vi "Aperture Server.vi"() -> ()   [LabVIEW 2018]
doc: "Use this VI to connect and control an unknown DC motor stage with the C-843. Select first if the connected stage is analog or PWM driven. The VI runs \"C843_Configuration_Setup.vi\" without moving any axis. It defines axis 1 to be \"DEFAULT_STAGE\" (analog) or \"DEFAULT_STAGE_P\" (PWM), which corresponds to no limit switches, no reference switch, and a position unit of 1 count. It reads the current velocity, the maximum allowed velocity, and the PID values of this stage type and sets the servo state to ON. Then it runs in a loop, reading the current position value, and giving the user the possibility to make relative moves in forward or backward direction, or to set velocity and PID values. Pressing the STOP button will send a STP command to the board, set the servo state to OFF and stop the VI."
uses:
  APERTURE EVENTS.ctl
  PI STAGE LIMITS.ctl
  PI APERTURE POSITION.ctl
  PI STAGE MAXIMUMS.ctl
  <vilib>/userdefined/High Color/IMAQdx.ctl
  <vilib>/vision/Image Controls.llb/Vision Info Type2.ctl
  <vilib>/Utility/miscctls.llb/LVMinMaxIncTypeDef.ctl
  <vilib>/Utility/Variable/NI_VariableUtilities.lvlib
  <vilib>/vision/NI_Vision_Development_Module.lvlib
  <vilib>/vision/driver/NI_Vision_Acquisition_Software.lvlib
panel:
  in  "ENABLE CAM":bool=TRUE
  in  "SET APERTURE":cluster{"Xm":dbl, "Ym":dbl} {"Ym" min=0.0 max=1.0 step=0.1 format="%.3f"; "Xm" min=0.0 max=12.5 step=0.1 format="%.3f"}
  in  "SET POSITION":T1 {"Yo" min=0.0 max=10.0 step=0.1 format="%.3f"; "Xo" min=0.0 max=12.5 step=0.1 format="%.3f"}
  out "APERTURE POSITION":cluster{"Xm":dbl, "Ym":dbl} {"Ym" format="%.3f"; "Xm" format="%.3f"}
  out "OBJECT POSITION":T1 {"Yo" format="%.3f"; "Xo" min=0.0 max=12.5 step=0.1 format="%.3f"}
  out "LIMITS ?":T2
  out "REFER?":T3
  out "ON TARG":T4
  out "SERVO?":T4
  out "HOMED":T5
  in  "INIT":bool=TRUE
  out "elements":T6[](array[typedef])
  in  "stop":bool
  in  "CLEAR ERRORS":bool
  out "PROCESS":string
  out "Identification":string
  out "Line Profile Graph":u8[](graph) caption="Line Profile"
  in  "Calibration Axis Info (Aperture Calibration)":T7={"Origin Pixel"={"X"=227.0, "Y"=1000.0}, "X Axis Pixel"={"X"=276.9972, "Y"=1000.52985}, "Axis Reference"=1} {"Axis Reference" items=["Direct", "Indirect"]}
  out "Image":T8(plugin-control)
  in  "PIXEL CALIBRATION":T9={"XSTEP SIZE"=5.7150000000000025, "YSTEP SIZE"=6.25, "UNITS"=2} {"UNITS" items=["Undefined", "Angstroms", "Microns"]; "YSTEP SIZE" format="%_4g"; "XSTEP SIZE" format="%_4g"}
  in  "BCG":T10={"BRIGHT"=150.0, "CONTRAST"=30.0, "GAMMA"=1.0} {"GAMMA" format="%_3f"}
  out "x-y":u16
  out "x*y":dbl
  in  "Tab Control":enum32{" SHIFTING", "SETTINGS", "RANGE"}(tab)
  out "HOMED":bool
  in  "AXIS":u16(ring) items=["1", "2", "3", "4"]
  in  "HOME LIMIT":enum16{"NEGATIVE", "POSITIVE"}(ring)
  in  "Stop":bool
  in  "STEP":dbl=1.0 min=0.0 max=1.0 step=0.1 format="%.4f"
  in  "OUT (+)":bool
  in  "IN (-)":bool
  in  "HOME":bool
  in  "HOME AXES":enum16{"1 & 2", "3 & 4"}(ring)
  out "Axis moving?":bool[](array[boolean])
  out "READY AXES":string[](array[string])
  in  "SERVO PID":cluster{"P":dbl, "I":dbl, "D":dbl}={"P"=140.0, "I"=14.0, "D"=300.0} {"P" format="%#.6f"; "I" format="%#.6f"; "D" format="%#.6f"}
  in  "STARTUP":T6[](array[typedef])=[enum."INIT PI CONTROLLER", enum."READ STAGE LIMIT SWITCHES ", enum."READ RON?", enum."SET SERVO MOTORS ON", enum."HOMED ?", enum."READ MIN POSITION: LIMIT OR SOFT"]
  in  "VELOCITY":dbl=10.0 format="%#.0p"
  out "STAGE MIN CLUSTER":T11 {"Xo MAX" format="%.6f"; "Xm MAX" format="%.6f"; "Ym MAX" format="%.6f"; "Yo MAX" format="%.6f"}
  out "STAGE MAX CLUSTER":T12 {"Xo MAX" format="%.6f"; "Xm MAX" format="%.6f"; "Ym MAX" format="%.6f"; "Yo MAX" format="%.6f"}
  in  "error in":errorcluster
  out "error out":errorcluster
  # "Radius 5.75cm for top element to\n centre optical element"
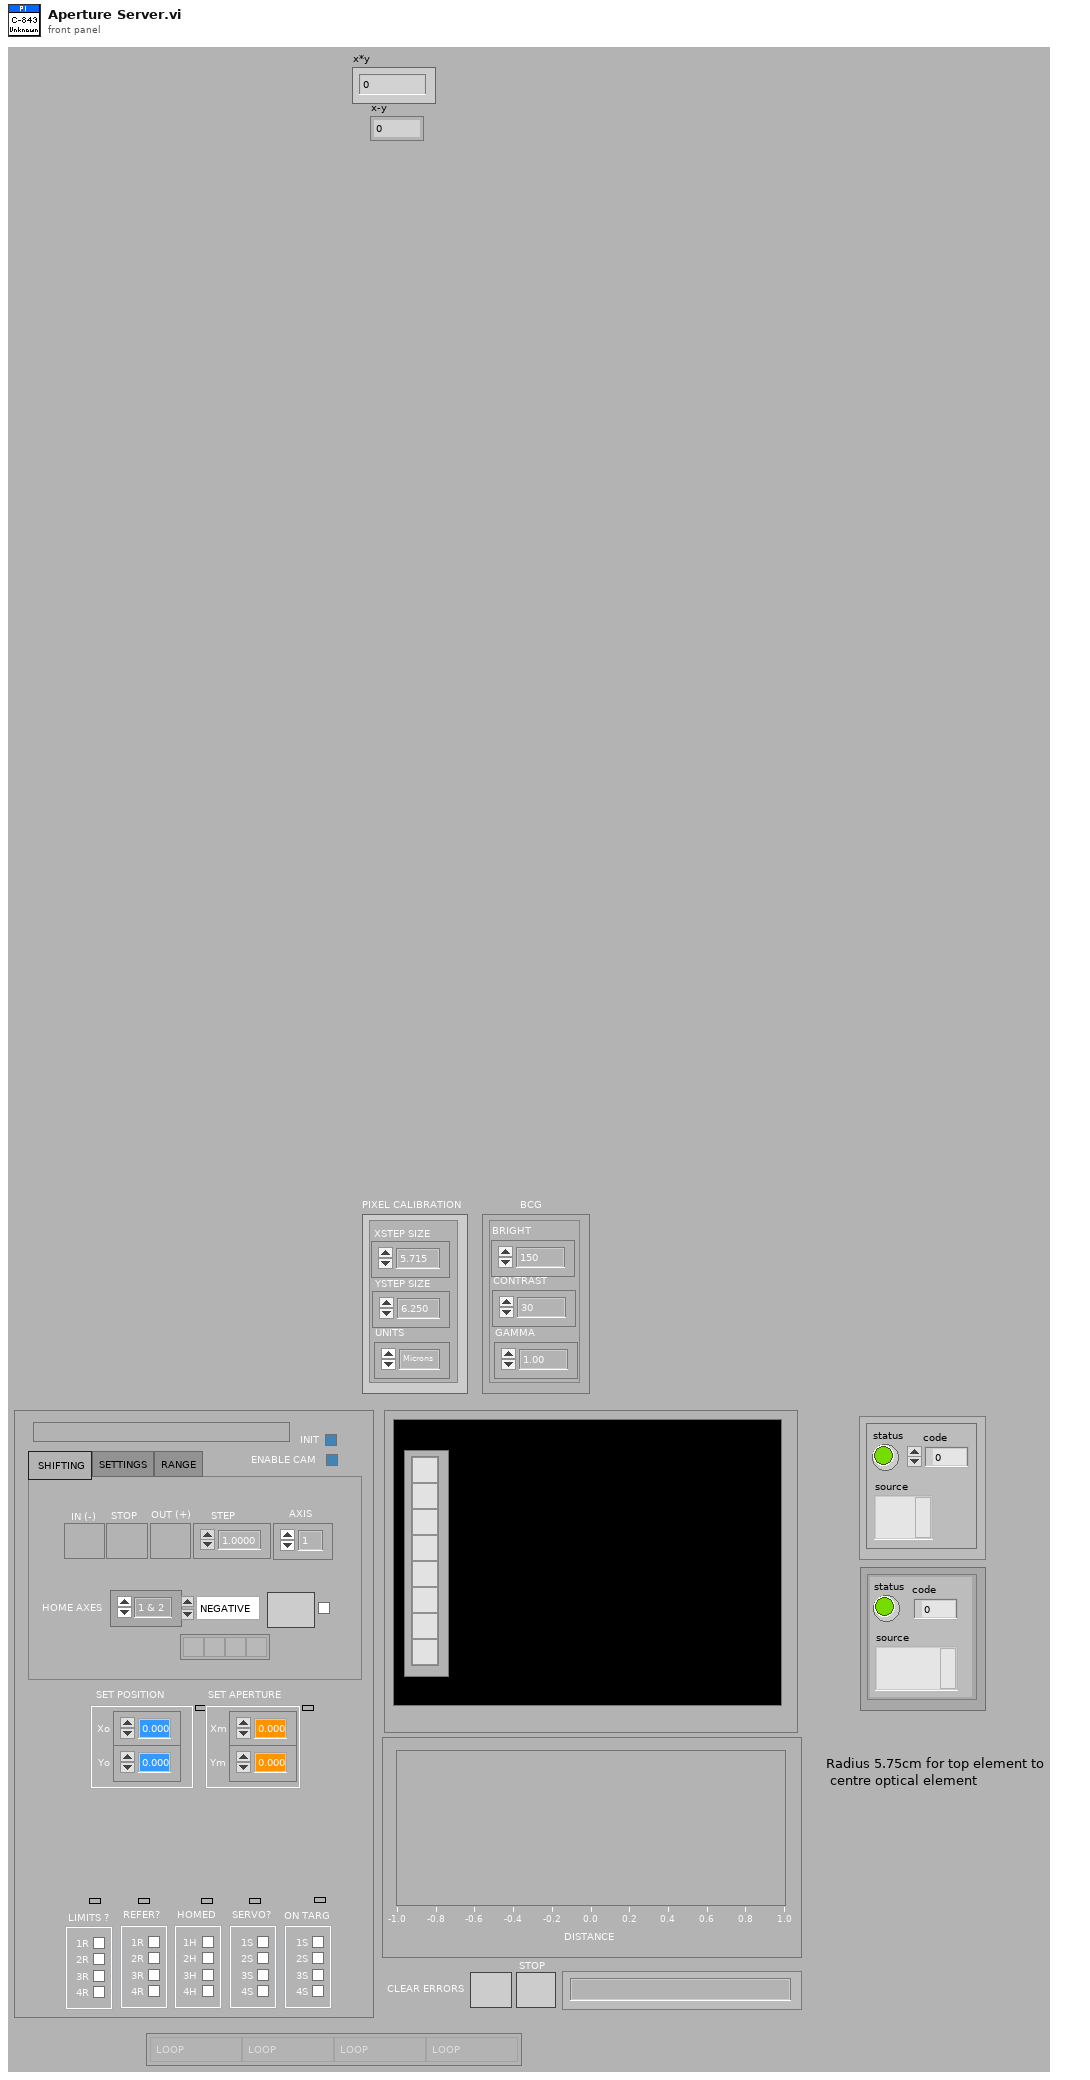
[diagram p1: front panel]
types:
  T1 = typedef "PI APERTURE POSITION.ctl" = cluster{"Xo":dbl, "Yo":dbl}
  T2 = typedef "PI STAGE LIMITS.ctl" = cluster{"1R":bool, "2R":bool, "3R":bool, "4R":bool}
  T3 = cluster{"1R":bool, "2R":bool, "3R":bool, "4R":bool}
  T4 = cluster{"1S":bool, "2S":bool, "3S":bool, "4S":bool}
  T5 = cluster{"1H":bool, "2H":bool, "3H":bool, "4H":bool}
  T6 = typedef "APERTURE EVENTS.ctl" = enum16{"LOOP", "INIT PI CONTROLLER", "WAIT FOR READY", "CLR ERRORS", "GOTO LIMIT", "HOMED ?", "READ MIN POSITION: LIMIT OR SOFT", "READ STAGE LIMIT SWITCHES ", "READ RON?", "GOTO POSITION", "SET POSITION", "GOTO LEFT", "GOTO RIGHT", "READ POSITION", "READ SERVO SETTINGS", "SET SERVO PID", "SET SERVO MOTORS ON", "SET VELOCITIES"}
  T7 = cluster{"Origin Pixel":cluster{"X":sgl, "Y":sgl}, "X Axis Pixel":cluster{"X":sgl, "Y":sgl}, "Axis Reference":u32}
  T8 = typedef "IMAQ Image.ctl" = refnum<image>
  T9 = cluster{"XSTEP SIZE":dbl, "YSTEP SIZE":dbl, "UNITS":u16}
  T10 = cluster{"BRIGHT":dbl, "CONTRAST":dbl, "GAMMA":dbl}
  T11 = typedef "PI STAGE MAXIMUMS.ctl" = cluster{"Xo MAX":dbl, "Xm MAX":dbl, "Yo MAX":dbl, "Ym MAX":dbl}
  T12 = cluster{"Xo MAX":dbl, "Xm MAX":dbl, "Yo MAX":dbl, "Ym MAX":dbl}
  T13 = typedef "IMAQdx.ctl" = refnum<k21>
  T14 = typedef "Vision Info Type2.ctl" = u32
  T15 = cluster{"Global Rectangle":i32[], "Contours":cluster{"Contour Type":u32, "ROI Type":u32, "Points":i32[]}[]}
  T16 = cluster{"Boolean":bool, "Boolean":bool, "Boolean":bool, "Boolean":bool}
  T17 = typedef "LVMinMaxIncTypeDef.ctl" = cluster{"Minimum":dbl, "Maximum":dbl, "Increment":dbl}
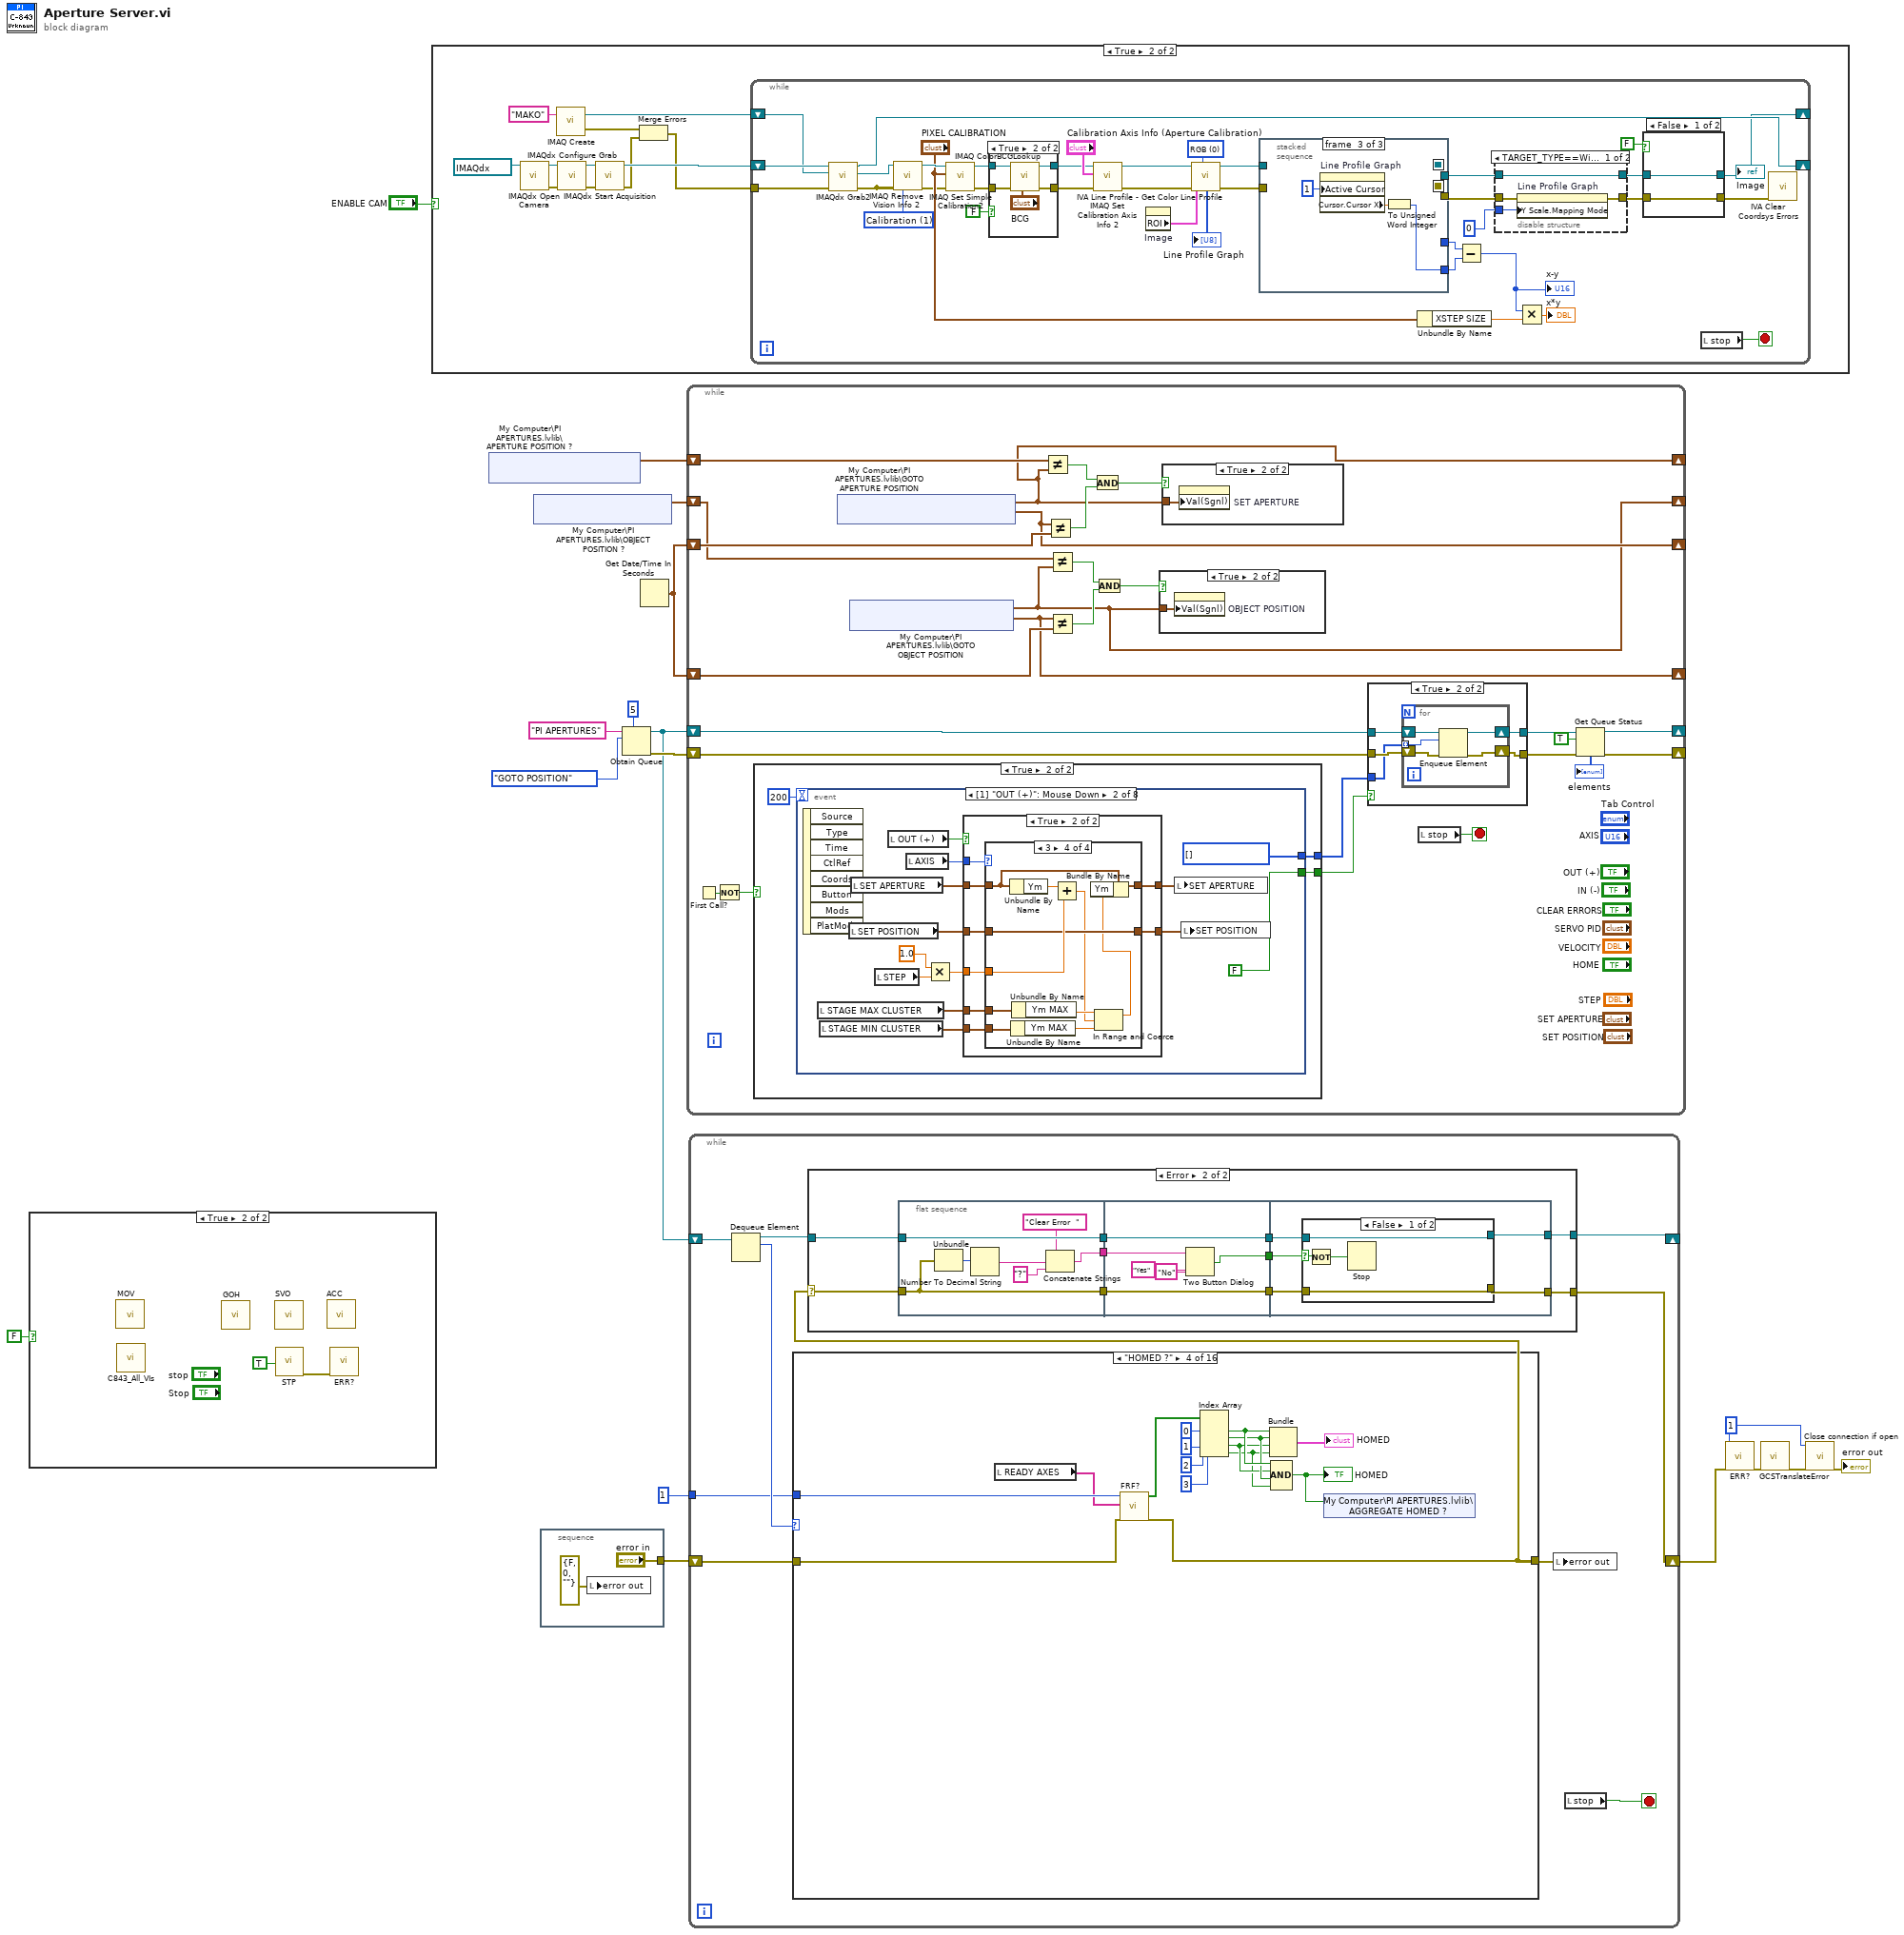
[diagram p0: block diagram]
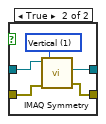
[diagram p3: hidden frame]
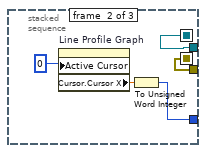
[diagram p6: hidden frame]
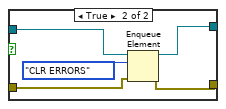
[diagram p10: hidden frame]
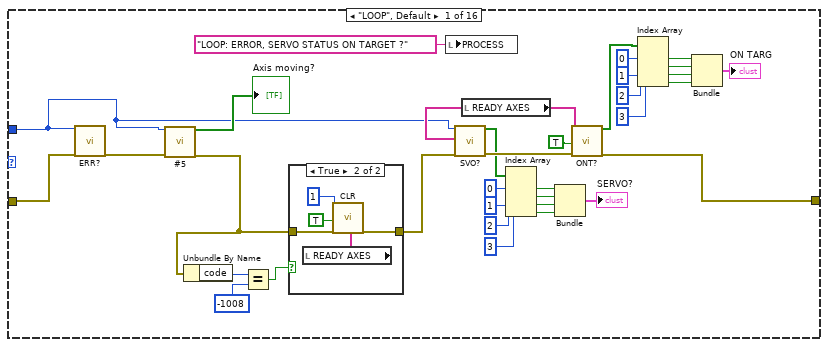
[diagram p11: hidden frame]
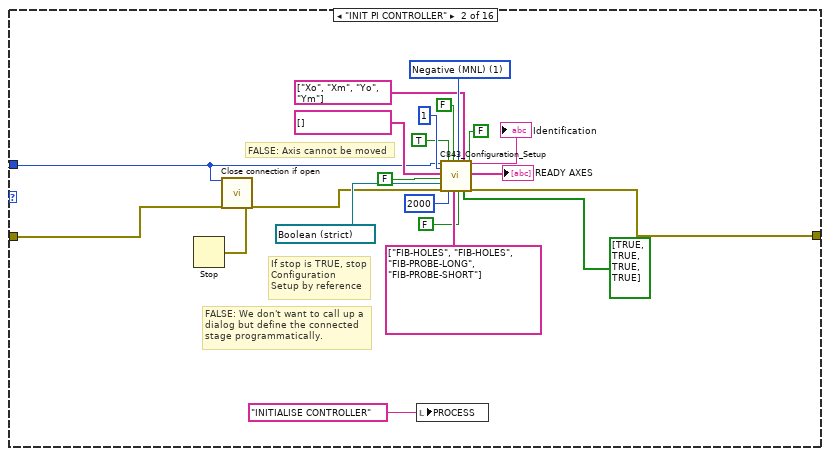
[diagram p13: hidden frame]
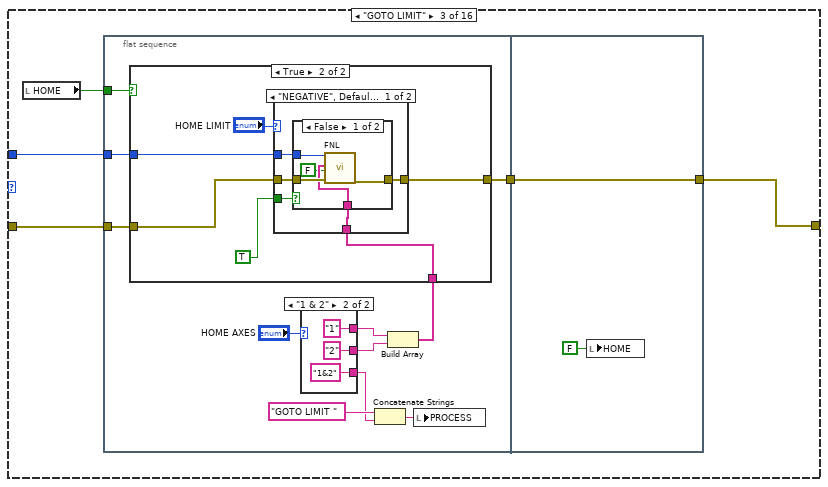
[diagram p14: hidden frame]
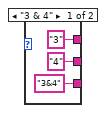
[diagram p15: hidden frame]
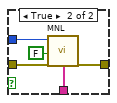
[diagram p17: hidden frame]
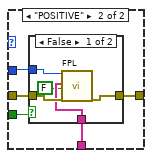
[diagram p18: hidden frame]
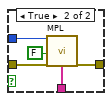
[diagram p19: hidden frame]
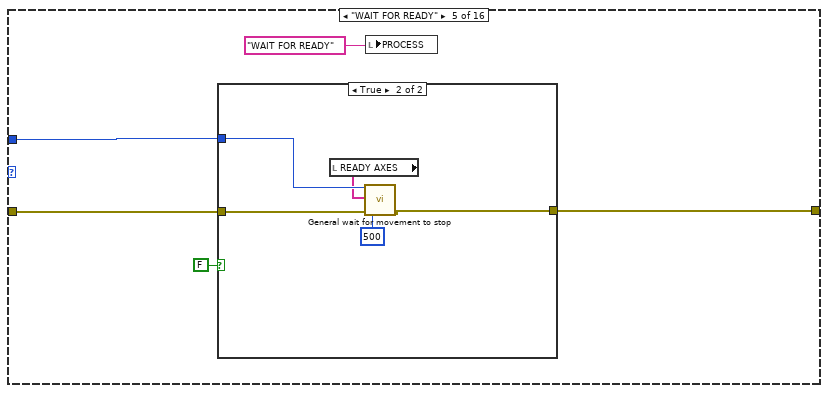
[diagram p20: hidden frame]
diagram:
  w5 = 1 ("System no.")
  n1 = case shown="True" FALSE {
    frame False {
    }
    frame True {
      n2 = call "MOV.vi"() -> ()  [unwired: 5 in, 15 out]
      n3 = call "C843_All_VIs.vi"() -> ()  [unwired: 1 in]
      n4 = call "GOH.vi"() -> ()  [unwired: 5 in, 15 out]
      n5 = call "SVO.vi"() -> ()  [unwired: 5 in, 15 out]
      n6 = call "STP.vi"("All axes?"=TRUE) -> ("error out"=w19:errorcluster)  [unwired: 4 in, 14 out]
      n7 = call "ACC.vi"() -> ()  [unwired: 6 in, 14 out]
      n8 = call "ERR?.vi"("error in"=w19) -> ()  [unwired: 1 in, 18 out]
    }
  }
  n9 = case shown="True" "ENABLE CAM" {
    frame False {
    }
    frame True {
      n10 = call <vilib>:"IMAQdx Open Camera.vi"("Session In"=T13 "MAKO") -> ("error out"=w27:errorcluster, "Session Out"=w29:T13)  [unwired: 9 in]
      n11 = call "IMAQ Create"("Image Name"="MAKO") -> ("New Image"=w23:T8, "error out"=w22:errorcluster)  [unwired: 4 in]
      n12 = call <vilib>:"IMAQdx Configure Grab.vi"("error in"=w27, "Session In"=w29) -> ("error out"=w26:errorcluster, "Session Out"=w28:T13)  [unwired: 8 in]
      n13 = call <vilib>:"IMAQdx Start Acquisition.vi"("error in"=w26, "Session In"=w28) -> ("error out"=w21:errorcluster, "Session Out"=w24:T13)  [unwired: 8 in]
      n14 = Merge Errors(w22, w21) -> (w20:errorcluster)
      n15 = while {
        tunnel: w20 -> [w43]
        shift-right: [w39] -> _
        shift-left: w24 -> [w42]
        shift-right: [w35] -> _
        shift-left: w23 -> [w38]
        stop <- w37 stop-if-true
        w63 = u16 0 items=["RGB", "HSL", "HSV", "HSI"] ("Color Mode")
        w66 = T14 1 items=["Any", "Calibration", "Overlay", "Grayscale Template", "Color Template", "Geometric Template", "Custom Data", "Golden Template", "Geometric Template 2", "Contour Data", "Camera Model"] ("Vision Info")
        n16 = call <vilib>:"IMAQdx Grab2.vi"("error in"=w43, "Image In"=w38, "Session In"=w42) -> ("error out"=w40:errorcluster, "Image Out"=w41:T8, "Session Out"=w39:T13)  [unwired: 5 in, 1 out]
        n17 = call "IMAQ Remove Vision Info 2"("error in (no error)"=w40, "Vision Info"=w66, "Image"=w41) -> ("Image Out"=w65:T8)  [unwired: 8 out]
        n18 = call "IMAQ Set Simple Calibration2"("error in (no error)"=w40, "Pixel Distances"="PIXEL CALIBRATION", "Image"=w65) -> ("error out"=w56:errorcluster, "Calibration Template Image"=w58:T8)  [unwired: 2 in, 5 out]
        n19 = case shown="True" FALSE {
          tunnel: w58 -> [w75 w80]
          tunnel: [w75 w79] -> w57
          tunnel: w56 -> [w74 w78]
          tunnel: [w74 w77] -> w55
          frame False {
          }
          frame True {
            n20 = call "IMAQ ColorBCGLookup"("Green BCG Values"="BCG", "error in (no error)"=w78, "Image Src"=w80) -> ("error out"=w77:errorcluster, "Image Dst Out"=w79:T8)  [unwired: 4 in, 3 out]
          }
        }
        n21 = call-poly "IMAQ Set Calibration Axis Info 2"("error in (no error)"=w55, "Calibration Axis Info"="Calibration Axis Info (Aperture Calibration)", "Calibration Template Image In"=w57) -> ("error out"=w61:errorcluster, "Calibration Template Image Out"=w62:T8)  [unwired: 7 out]
        n22 = property on="Image" class="ImageControl"() -> ("ROI"=w54:T15)  [unwired: 2 in, 2 out]
        n23 = call <vilib>:"IVA Line Profile - Get Color Line Profile.vi"("Color Mode"=w63, "error in (no error)"=w61, "ROI Descriptor"=w54, "Image In"=w62) -> ("error out"=w50:errorcluster, "Green or Sat Pixels"=→"Line Profile Graph":u8[], "Image Out"=w52:T8)  [unwired: 5 out]
        n24 = stacked-sequence {
          seq-local: [w82 _ _] -> [_ w84 _]
          seq-local: [w81 _ _] -> [_ w83 _]
          tunnel: w52 -> [w82 _ _]
          tunnel: w50 -> [w81 _ _]
          tunnel: [_ w84 _] -> w53
          tunnel: [_ w83 _] -> w51
          tunnel: [_ w85 _] -> w49
          tunnel: [_ _ w88] -> w48
          frame #0 {
          }
          frame #1 {
            n25 = property on="Line Profile Graph" class="WFGraph (strict)"("Active Cursor"=u32 0) -> ("Cursor.Cursor X"=w86:dbl)  [unwired: 2 in, 2 out]
            n26 = To Unsigned Word Integer(number=w86) -> (unsigned 16bit integer=w85:u16)
          }
          frame #2 {
            n27 = property on="Line Profile Graph" class="WFGraph (strict)"("Active Cursor"=u32 1) -> ("Cursor.Cursor X"=w89:dbl)  [unwired: 2 in, 2 out]
            n28 = To Unsigned Word Integer(number=w89) -> (unsigned 16bit integer=w88:u16)
          }
        }
        n29 = Unbundle By Name("PIXEL CALIBRATION") -> ("XSTEP SIZE"=w45:dbl)
        n30 = Subtract(x=w49, y=w48) -> (x-y=w47:u16)
        "x-y" <- w47
        n31 = disable-structure "Conditional Disable Structure" shown="TARGET_TYPE==Windows" {
          disable-tunnel: w51 -> [w94 w95]
          disable-tunnel: [w93 w95] -> w33
          disable-tunnel: w53 -> [w92 w96]
          disable-tunnel: [w92 w96] -> w34
          disable-tunnel: u8 0 ("Y Scale.Mapping Mode") -> [w91 _]
          frame condition #0 (active) {
            n32 = property on="Line Profile Graph" class="WFGraph (strict)"(error in=w94, "Y Scale.Mapping Mode"=w91) -> (error out=w93:errorcluster)  [unwired: 1 in, 1 out]
          }
          frame condition #1 {
          }
        }
        n33 = Multiply(x=w47, y=w45) -> (x*y=→"x*y":dbl)
        n34 = case shown="False" FALSE {
          tunnel: [w68 w73] -> w35
          tunnel: w34 -> [w68 w72]
          tunnel: w33 -> [w67 w70]
          tunnel: [w67 w69] -> w32
          frame False {
          }
          frame True {
            w71 = u32 1 items=["Horizontal", "Vertical", "Central", "1st Diagonal", "2nd Diagonal"] ("Type of Symmetry")
            n35 = call "IMAQ Symmetry"("error in (no error)"=w70, "Type of Symmetry"=w71, "Image Src"=w72) -> ("error out"=w69:errorcluster, "Image Dst Out"=w73:T8)  [unwired: 2 in]
          }
        }
        "Image" <- w35
        n36 = local read "stop"() -> (w37:bool)
        n37 = call <vilib>:"IVA Clear Coordsys Errors.vi"("error in (no error)"=w32) -> ()  [unwired: 10 in, 1 out]
      }
    }
  }
  n38 = shared-variable "My Computer\\PI APERTURES.lvlib\\APERTURE POSITION ?"() -> (w3:cluster{"Xm":dbl, "Ym":dbl})  [unwired: 1 in, 2 out]
  n39 = shared-variable "My Computer\\PI APERTURES.lvlib\\OBJECT POSITION ?"() -> (w2:cluster{"Xm":dbl, "Ym":dbl})  [unwired: 1 in, 2 out]
  n40 = stacked-sequence {
    tunnel: ["error in"] -> w6
    frame #0 {
      n41 = local write "error out"(errorcluster {"status"=FALSE, "code"=0, "source"=""} ("error in")) -> ()
    }
  }
  n42 = Obtain Queue(max queue size (-1, unlimited)=5, name (unnamed)="PI APERTURES", element data type=APERTURE_EVENTS."GOTO POSITION") -> (queue out=w11:refnum<queue>, error out=w12:errorcluster)  [unwired: 2 in, 1 out]
  n43 = Get Date/Time In Seconds() -> (seconds since 1Jan1904=w4:timestamp)
  n44 = while {
    shift-right: [w119] -> _
    shift-left: w11 -> [w115]
    shift-right: [w117] -> _
    shift-left: w12 -> [w114]
    shift-right: [w111] -> _
    shift-left: w4 -> [w112]
    shift-right: [w109] -> _
    shift-left: w4 -> [w110]
    shift-right: [w100] -> _
    shift-left: w3 -> [w105]
    shift-right: [w99] -> _
    shift-left: w2 -> [w104]
    stop <- w121 stop-if-true
    n45 = First Call?() -> (First Call?: T/F=w123:bool)
    n46 = Not(x=w123) -> (.not. x?=w122:bool)
    n47 = case shown="True" w122 {
      tunnel: [w133 w141] -> w125
      tunnel: [TRUE w140] -> w124
      frame False {
        n48 = local write "HOME AXES"(enum16{"1 & 2", "3 & 4"}."1 & 2" ("HOME AXES")) -> ()
        n49 = local write "HOME LIMIT"(enum16{"NEGATIVE", "POSITIVE"}."NEGATIVE" ("HOME LIMIT")) -> ()
        n50 = Delete From Array(array="STARTUP", length=1, index=0) -> (array with subset deleted=w132:T6[])  [unwired: 1 out]
        n51 = case shown="False" "INIT" {
          tunnel: [w138 w139] -> w133
          tunnel: w132 -> [w138 _]
          tunnel: "STARTUP" -> [_ w139]
          frame False {
          }
          frame True {
          }
        }
        "PROCESS" <- "" ("PROCESS")
      }
      frame True {
        n52 = event shown="[1] \"OUT (+)\": Mouse Down" {
          selector: _ -> [_ _ _ _ _ _ _ _]
          dyn-events: _ -> [_ _ _ _ _ _ _ _]
          timeout: 200 -> [_ _ _ _ _ _ _ _]
          tunnel: [w144 w149 w216 w280 w282 w284 w285 w288] -> w141
          tunnel: [TRUE FALSE ("HOMED") FALSE ("HOMED") w279 TRUE TRUE TRUE TRUE] -> w140
          event Timeout {
            w144 = T6[] [enum."LOOP", enum."READ POSITION", enum."HOMED ?"] items=["LOOP", "INIT PI CONTROLLER", "WAIT FOR READY", "CLR ERRORS", "GOTO LIMIT", "HOMED ?", "READ MIN POSITION: LIMIT OR SOFT", "READ STAGE LIMIT SWITCHES ", "READ RON?", "GOTO POSITION", "SET POSITION", "GOTO LEFT", "GOTO RIGHT", "READ POSITION", "READ SERVO SETTINGS", "SET SERVO PID", "SET SERVO MOTORS ON", "SET VELOCITIES"]
            n53 = event-data() -> ()  [unwired: 1 in, 3 out]
            n54 = call <vilib>:"Flush Shared Variable Data.vi"() -> ()  [unwired: 11 in, 1 out]
          }
          event "OUT (+)": Mouse Down {
            w149 = T6[] [] items=["LOOP", "INIT PI CONTROLLER", "WAIT FOR READY", "CLR ERRORS", "GOTO LIMIT", "HOMED ?", "READ MIN POSITION: LIMIT OR SOFT", "READ STAGE LIMIT SWITCHES ", "READ RON?", "GOTO POSITION", "SET POSITION", "GOTO LEFT", "GOTO RIGHT", "READ POSITION", "READ SERVO SETTINGS", "SET SERVO PID", "SET SERVO MOTORS ON", "SET VELOCITIES"]
            n55 = event-data() -> ()  [unwired: 1 in, 8 out]
            n56 = local read "STAGE MAX CLUSTER"() -> (w145:T12)
            n57 = local read "STAGE MIN CLUSTER"() -> (w146:T11)
            n58 = local read "SET POSITION"() -> (w155:T1)
            n59 = local read "SET APERTURE"() -> (w156:cluster{"Xm":dbl, "Ym":dbl})
            n60 = local read "STEP"() -> (w154:dbl)
            n61 = local read "OUT (+)"() -> (w147:bool)
            n62 = local read "AXIS"() -> (w153:u16)
            n63 = Multiply(x=1.0, y=w154) -> (x*y=w157:dbl)
            n64 = case shown="True" w147 {
              tunnel: w157 -> [_ w167]
              tunnel: w156 -> [w159 w166]
              tunnel: w155 -> [w158 w165]
              tunnel: w153 -> [_ w164]
              tunnel: [w158 w163] -> w151
              tunnel: [w159 w162] -> w150
              tunnel: w146 -> [_ w161]
              tunnel: w145 -> [_ w160]
              frame False {
              }
              frame True {
                n65 = case shown="3" w164 {
                  tunnel: w165 -> [w176 w187 w198 w207]
                  tunnel: w166 -> [w174 w188 w196 w210]
                  tunnel: w167 -> [w177 w185 w199 w208]
                  tunnel: [w175 w187 w197 w207] -> w163
                  tunnel: [w174 w186 w196 w209] -> w162
                  tunnel: w161 -> [w172 w181 w192 w201]
                  tunnel: w160 -> [w173 w182 w193 w202]
                  frame 0, Default {
                    n66 = Unbundle By Name(w172) -> ("Xo MAX"=w170:dbl)
                    n67 = Unbundle By Name(w173) -> ("Xo MAX"=w171:dbl)
                    n68 = Unbundle By Name(w176) -> ("Xo"=w178:dbl)
                    n69 = Add(x=w178, y=w177) -> (x+y=w169:dbl)
                    n70 = In Range and Coerce(upper limit=w171, x=w169, lower limit=w170) -> (coerced(x)=w168:dbl)  [unwired: 1 out]
                    n71 = Bundle By Name(cluster=w176, "Xo"=w168) -> (w175:T1)
                  }
                  frame 1 {
                    n72 = Unbundle By Name(w188) -> ("Xm"=w189:dbl)
                    n73 = Unbundle By Name(w181) -> ("Xm MAX"=w183:dbl)
                    n74 = Unbundle By Name(w182) -> ("Xm MAX"=w184:dbl)
                    n75 = Add(x=w189, y=w185) -> (x+y=w180:dbl)
                    n76 = In Range and Coerce(upper limit=w184, x=w180, lower limit=w183) -> (coerced(x)=w179:dbl)  [unwired: 1 out]
                    n77 = Bundle By Name(cluster=w188, "Xm"=w179) -> (w186:cluster{"Xm":dbl, "Ym":dbl})
                  }
                  frame 2 {
                    n78 = Unbundle By Name(w192) -> ("Yo MAX"=w195:dbl)
                    n79 = Unbundle By Name(w193) -> ("Yo MAX"=w194:dbl)
                    n80 = Unbundle By Name(w198) -> ("Yo"=w200:dbl)
                    n81 = Add(x=w200, y=w199) -> (x+y=w191:dbl)
                    n82 = In Range and Coerce(upper limit=w194, x=w191, lower limit=w195) -> (coerced(x)=w190:dbl)  [unwired: 1 out]
                    n83 = Bundle By Name(cluster=w198, "Yo"=w190) -> (w197:T1)
                  }
                  frame 3 {
                    n84 = Unbundle By Name(w210) -> ("Ym"=w211:dbl)
                    n85 = Unbundle By Name(w201) -> ("Ym MAX"=w206:dbl)
                    n86 = Unbundle By Name(w202) -> ("Ym MAX"=w205:dbl)
                    n87 = Add(x=w211, y=w208) -> (x+y=w204:dbl)
                    n88 = In Range and Coerce(upper limit=w205, x=w204, lower limit=w206) -> (coerced(x)=w203:dbl)  [unwired: 1 out]
                    n89 = Bundle By Name(cluster=w210, "Ym"=w203) -> (w209:cluster{"Xm":dbl, "Ym":dbl})
                  }
                }
              }
            }
            n90 = local write "SET APERTURE"(w150) -> ()
            n91 = local write "SET POSITION"(w151) -> ()
          }
          event "IN (-)": Mouse Down {
            w216 = T6[] [] items=["LOOP", "INIT PI CONTROLLER", "WAIT FOR READY", "CLR ERRORS", "GOTO LIMIT", "HOMED ?", "READ MIN POSITION: LIMIT OR SOFT", "READ STAGE LIMIT SWITCHES ", "READ RON?", "GOTO POSITION", "SET POSITION", "GOTO LEFT", "GOTO RIGHT", "READ POSITION", "READ SERVO SETTINGS", "SET SERVO PID", "SET SERVO MOTORS ON", "SET VELOCITIES"]
            n92 = event-data() -> ()  [unwired: 1 in, 7 out]
            n93 = local read "STAGE MAX CLUSTER"() -> (w212:T12)
            n94 = local read "STAGE MIN CLUSTER"() -> (w213:T11)
            n95 = local read "SET POSITION"() -> (w222:T1)
            n96 = local read "SET APERTURE"() -> (w223:cluster{"Xm":dbl, "Ym":dbl})
            n97 = local read "STEP"() -> (w221:dbl)
            n98 = local read "OUT (+)"() -> (w214:bool)
            n99 = local read "AXIS"() -> (w220:u16)
            n100 = Multiply(x=-1.0, y=w221) -> (x*y=w224:dbl)
            n101 = case shown="True" w214 {
              tunnel: w224 -> [_ w234]
              tunnel: w223 -> [w226 w233]
              tunnel: w222 -> [w225 w232]
              tunnel: w220 -> [_ w231]
              tunnel: [w225 w230] -> w218
              tunnel: [w226 w229] -> w217
              tunnel: w213 -> [_ w228]
              tunnel: w212 -> [_ w227]
              frame False {
              }
              frame True {
                n102 = case shown="3" w231 {
                  tunnel: w232 -> [w243 w254 w265 w274]
                  tunnel: w233 -> [w241 w255 w263 w277]
                  tunnel: w234 -> [w244 w252 w266 w275]
                  tunnel: [w242 w254 w264 w274] -> w230
                  tunnel: [w241 w253 w263 w276] -> w229
                  tunnel: w228 -> [w239 w248 w259 w268]
                  tunnel: w227 -> [w240 w249 w260 w269]
                  frame 0, Default {
                    n103 = Unbundle By Name(w240) -> ("Xo MAX"=w238:dbl)
                    n104 = Unbundle By Name(w239) -> ("Xo MAX"=w237:dbl)
                    n105 = Unbundle By Name(w243) -> ("Xo"=w245:dbl)
                    n106 = Add(x=w245, y=w244) -> (x+y=w236:dbl)
                    n107 = In Range and Coerce(upper limit=w238, x=w236, lower limit=w237) -> (coerced(x)=w235:dbl)  [unwired: 1 out]
                    n108 = Bundle By Name(cluster=w243, "Xo"=w235) -> (w242:T1)
                  }
                  frame 1 {
                    n109 = Unbundle By Name(w255) -> ("Xm"=w256:dbl)
                    n110 = Unbundle By Name(w248) -> ("Xm MAX"=w250:dbl)
                    n111 = Unbundle By Name(w249) -> ("Xm MAX"=w251:dbl)
                    n112 = Add(x=w256, y=w252) -> (x+y=w247:dbl)
                    n113 = In Range and Coerce(upper limit=w251, x=w247, lower limit=w250) -> (coerced(x)=w246:dbl)  [unwired: 1 out]
                    n114 = Bundle By Name(cluster=w255, "Xm"=w246) -> (w253:cluster{"Xm":dbl, "Ym":dbl})
                  }
                  frame 2 {
                    n115 = Unbundle By Name(w259) -> ("Yo MAX"=w262:dbl)
                    n116 = Unbundle By Name(w260) -> ("Yo MAX"=w261:dbl)
                    n117 = Unbundle By Name(w265) -> ("Yo"=w267:dbl)
                    n118 = Add(x=w267, y=w266) -> (x+y=w258:dbl)
                    n119 = In Range and Coerce(upper limit=w261, x=w258, lower limit=w262) -> (coerced(x)=w257:dbl)  [unwired: 1 out]
                    n120 = Bundle By Name(cluster=w265, "Yo"=w257) -> (w264:T1)
                  }
                  frame 3 {
                    n121 = Unbundle By Name(w268) -> ("Ym MAX"=w273:dbl)
                    n122 = Unbundle By Name(w269) -> ("Ym MAX"=w272:dbl)
                    n123 = Unbundle By Name(w277) -> ("Ym"=w278:dbl)
                    n124 = Add(x=w278, y=w275) -> (x+y=w271:dbl)
                    n125 = In Range and Coerce(upper limit=w272, x=w271, lower limit=w273) -> (coerced(x)=w270:dbl)  [unwired: 1 out]
                    n126 = Bundle By Name(cluster=w277, "Ym"=w270) -> (w276:cluster{"Xm":dbl, "Ym":dbl})
                  }
                }
              }
            }
            n127 = local write "SET APERTURE"(w217) -> ()
            n128 = local write "SET POSITION"(w218) -> ()
          }
          event "SET APERTURE": Value Change {
            w280 = T6[] [enum."GOTO POSITION"] items=["LOOP", "INIT PI CONTROLLER", "WAIT FOR READY", "CLR ERRORS", "GOTO LIMIT", "HOMED ?", "READ MIN POSITION: LIMIT OR SOFT", "READ STAGE LIMIT SWITCHES ", "READ RON?", "GOTO POSITION", "SET POSITION", "GOTO LEFT", "GOTO RIGHT", "READ POSITION", "READ SERVO SETTINGS", "SET SERVO PID", "SET SERVO MOTORS ON", "SET VELOCITIES"]
            n129 = event-data() -> ()  [unwired: 1 in, 3 out]
            n130 = local read "HOMED"() -> (w279:bool)
          }
          event "CLEAR ERRORS": Mouse Down {
            w282 = T6[] [enum."CLR ERRORS", enum."WAIT FOR READY"] items=["LOOP", "INIT PI CONTROLLER", "WAIT FOR READY", "CLR ERRORS", "GOTO LIMIT", "HOMED ?", "READ MIN POSITION: LIMIT OR SOFT", "READ STAGE LIMIT SWITCHES ", "READ RON?", "GOTO POSITION", "SET POSITION", "GOTO LEFT", "GOTO RIGHT", "READ POSITION", "READ SERVO SETTINGS", "SET SERVO PID", "SET SERVO MOTORS ON", "SET VELOCITIES"]
            n131 = event-data() -> ()  [unwired: 1 in, 3 out]
          }
          event "HOME": Value Change {
            w284 = T6[] [enum."GOTO LIMIT", enum."CLR ERRORS", enum."HOMED ?"] items=["LOOP", "INIT PI CONTROLLER", "WAIT FOR READY", "CLR ERRORS", "GOTO LIMIT", "HOMED ?", "READ MIN POSITION: LIMIT OR SOFT", "READ STAGE LIMIT SWITCHES ", "READ RON?", "GOTO POSITION", "SET POSITION", "GOTO LEFT", "GOTO RIGHT", "READ POSITION", "READ SERVO SETTINGS", "SET SERVO PID", "SET SERVO MOTORS ON", "SET VELOCITIES"]
            n132 = event-data() -> ()  [unwired: 1 in, 3 out]
          }
          event "SERVO PID": Value Change {
            w285 = T6[] [enum."SET SERVO PID"] items=["LOOP", "INIT PI CONTROLLER", "WAIT FOR READY", "CLR ERRORS", "GOTO LIMIT", "HOMED ?", "READ MIN POSITION: LIMIT OR SOFT", "READ STAGE LIMIT SWITCHES ", "READ RON?", "GOTO POSITION", "SET POSITION", "GOTO LEFT", "GOTO RIGHT", "READ POSITION", "READ SERVO SETTINGS", "SET SERVO PID", "SET SERVO MOTORS ON", "SET VELOCITIES"]
            n133 = event-data() -> ()  [unwired: 1 in, 6 out]
          }
          event "VELOCITY": Value Change {
            w288 = T6[] [enum."SET VELOCITIES"] items=["LOOP", "INIT PI CONTROLLER", "WAIT FOR READY", "CLR ERRORS", "GOTO LIMIT", "HOMED ?", "READ MIN POSITION: LIMIT OR SOFT", "READ STAGE LIMIT SWITCHES ", "READ RON?", "GOTO POSITION", "SET POSITION", "GOTO LEFT", "GOTO RIGHT", "READ POSITION", "READ SERVO SETTINGS", "SET SERVO PID", "SET SERVO MOTORS ON", "SET VELOCITIES"]
            n134 = event-data() -> ()  [unwired: 1 in, 6 out]
          }
        }
      }
    }
    n135 = shared-variable "My Computer\\PI APERTURES.lvlib\\GOTO APERTURE POSITION"() -> (w100:cluster{"Xm":dbl, "Ym":dbl}, w111:timestamp)  [unwired: 1 in, 1 out]
    n136 = shared-variable "My Computer\\PI APERTURES.lvlib\\GOTO OBJECT POSITION"() -> (w99:cluster{"Xm":dbl, "Ym":dbl}, w109:timestamp)  [unwired: 1 in, 1 out]
    n137 = Not Equal?(x=w105, y=w100) -> (x != y?=w106:bool)
    n138 = Not Equal?(x=w111, y=w112) -> (x != y?=w107:bool)
    n139 = Not Equal?(x=w104, y=w99) -> (x != y?=w103:bool)
    n140 = Not Equal?(x=w109, y=w110) -> (x != y?=w102:bool)
    n141 = And(x=w106, y=w107) -> (x .and. y?=w108:bool)
    n142 = And(x=w103, y=w102) -> (x .and. y?=w101:bool)
    n143 = case shown="True" w101 {
      tunnel: w99 -> [_ w126]
      frame False {
      }
      frame True {
        n144 = property on="OBJECT POSITION" class="Clust (strict)"("Val(Sgnl)"=w126) -> ()  [unwired: 2 in, 2 out]
      }
    }
    n145 = case shown="True" w108 {
      tunnel: w100 -> [_ w127]
      frame False {
      }
      frame True {
        n146 = property on="SET APERTURE" class="Clust (strict)"("Val(Sgnl)"=w127) -> ()  [unwired: 2 in, 2 out]
      }
    }
    n147 = case shown="True" w124 {
      tunnel: w115 -> [w290 w295]
      tunnel: [w290 w294] -> w120
      tunnel: [w289 w293] -> w118
      tunnel: w114 -> [w289 w292]
      tunnel: w125 -> [_ w291]
      frame False {
      }
      frame True {
        n148 = for {
          shift-right: [w298] -> w294
          shift-left: w295 -> [w300]
          shift-right: [w297] -> w293
          shift-left: w292 -> [w299]
          tunnel: w291 -> [w296] mode=indexing
          n149 = Enqueue Element(queue=w300, element=w296, error in (no error)=w299) -> (queue out=w298:refnum<queue>, error out=w297:errorcluster)  [unwired: 1 in, 1 out]
        }
      }
    }
    n150 = local read "stop"() -> (w121:bool)
    n151 = Get Queue Status(queue=w120, return elements? (F)=TRUE, error in (no error)=w118) -> (queue out=w119:refnum<queue>, error out=w117:errorcluster, elements=→"elements":T6[])  [unwired: 5 out]
  }
  n152 = while {
    shift-right: [w302] -> _
    shift-left: w11 -> [w309]
    tunnel: 1 -> [w306]
    shift-right: [w301] -> w8
    shift-left: w6 -> [w305]
    stop <- w307 stop-if-true
    n153 = Dequeue Element(queue=w309) -> (queue out=w303:refnum<queue>, element=w308:T6)  [unwired: 2 in, 2 out]
    n154 = case shown="\"HOMED ?\"" w308 {
      tunnel: w306 -> [w349 w393 w413 w484 w487 w509 w533 w549 w559 w583 w613 w643 w662 w672 w678 w683]
      tunnel: w305 -> [w382 w397 w411 w482 w489 w508 w535 w548 w561 w582 w612 w642 w664 w673 w676 w685]
      tunnel: [w381 w389 w412 w481 w488 w506 w529 w547 w560 w577 w611 w641 w663 w671 w677 w684] -> w304
      frame "LOOP", Default {
        n155 = call "ERR?.vi"("System no."=w349, "error in"=w382) -> ("error out"=w352:errorcluster)  [unwired: 17 out]
        n156 = call "#5.vi"("System no."=w349, "error in"=w352) -> ("Axis moving?"=→"Axis moving?":bool[], "error out"=w351:errorcluster)  [unwired: 16 out]
        n157 = Unbundle By Name(w351) -> ("code"=w378:i32)
        n158 = Equal?(x=w378, y=-1008) -> (x = y?=w377:bool)
        n159 = case shown="True" w377 {
          tunnel: [w383 w385] -> w375
          tunnel: w351 -> [w383 w384]
          frame False {
          }
          frame True {
            n160 = local read "READY AXES"() -> (w387:string[])
            n161 = call "CLR.vi"("System no."=1, "CLR axes"=w387, "All axes?"=TRUE, "error in"=w384) -> ("error out"=w385:errorcluster)  [unwired: 1 in, 14 out]
          }
        }
        n162 = local write "PROCESS"("LOOP: ERROR, SERVO STATUS ON TARGET ?" ("PROCESS")) -> ()
        n163 = local read "READY AXES"() -> (w376:string[])
        n164 = call "SVO?.vi"("System no."=w349, "Axes to query"=w376, "error in"=w375) -> ("Servo status?"=w364:bool[], "error out"=w374:errorcluster)  [unwired: 2 in, 13 out]
        n165 = Index Array(array=w364, index #1=0 ("index"), index #2=1 ("index"), index #3=2 ("index"), index #4=3 ("index")) -> (element #1=w368:bool, element #2=w367:bool, element #3=w366:bool, element #4=w365:bool)
        n166 = Bundle("Boolean"=w368, "Boolean"=w367, "Boolean"=w366, "Boolean"=w365) -> (→"SERVO?":T16)  [unwired: 1 in]
        n167 = call "ONT?.vi"("Axes to query"=w376, "All axes?"=TRUE, "error in"=w374) -> ("Axis on target?"=w354:bool[], "error out"=w381:errorcluster)  [unwired: 2 in, 13 out]
        n168 = Index Array(array=w354, index #1=0 ("index"), index #2=1 ("index"), index #3=2 ("index"), index #4=3 ("index")) -> (element #1=w358:bool, element #2=w357:bool, element #3=w356:bool, element #4=w355:bool)
        n169 = Bundle("Boolean"=w358, "Boolean"=w357, "Boolean"=w356, "Boolean"=w355) -> (→"ON TARG":T16)  [unwired: 1 in]
      }
      frame "INIT PI CONTROLLER" {
        w405 = u16 1 items=["Positive (MPL)", "Negative (MNL)"] ("Limit switch selection")
        # "If stop is TRUE, stop \nConfiguration\nSetup by reference"
        # "FALSE: We don't want to call up a \ndialog but define the connected\nstage programmatically."
        # "FALSE: Axis cannot be moved"
        n170 = call "Close connection if open.vi"("System no."=w393, "error in"=w397) -> ("error out"=w396:errorcluster)  [unwired: 16 in, 1 out]
        n171 = Stop(stop? (T)=w396) -> ()
        n172 = local write "PROCESS"("INITIALISE CONTROLLER" ("PROCESS")) -> ()
        n173 = call "C843_Configuration_Setup.vi"("System no."=w393, "C-843 Board No."=1, "Axes to move"=string[] [], "All axes?"=FALSE, "Stop refnum"=refnum<vi> refnum, "error in"=w396, "C-843 version"=TRUE, "Timeout"=u32 2000, "Use dialog to define\nconnected stages?"=FALSE ("Use dialog to define\nconnected stages?"), "Stage names input"=string[] ["FIB-HOLES", "FIB-HOLES", "FIB-PROBE-LONG", "FIB-PROBE-SHORT"], "Limit switch selection"=w405, "Define home?"=FALSE, "RON Affected axes"=string[] ["Xo", "Xm", "Yo", "Ym"], "Reference mode"=bool[] [TRUE, TRUE, TRUE, TRUE], "Move to middle?"=FALSE) -> ("Identification"=→"Identification":string, "Conn. \nAxes"=→"READY AXES":string[], "error out"=w389:errorcluster)  [unwired: 2 out]
      }
      frame "GOTO LIMIT" {
        n174 = local read "HOME"() -> (w410:bool)
        n175 = flat-sequence {
          tunnel: w413 -> [w424]
          tunnel: w411 -> [w422]
          tunnel: w410 -> [w421]
          tunnel: [w423] -> w409
          tunnel: [w469] -> w412
          tunnel: w409 -> [w469]
          frame #0 {
            n176 = case shown="\"1 & 2\"" "HOME AXES" {
              tunnel: ["3" "1"] -> w416
              tunnel: ["4" "2"] -> w415
              tunnel: ["3&4" "1&2"] -> w414
              frame "3 & 4" {
              }
              frame "1 & 2" {
              }
            }
            n177 = Concatenate Strings("GOTO LIMIT ", w414) -> (w418:string)
            n178 = Build Array(w416, w415) -> (w420:string[])
            n179 = case shown="True" w421 {
              tunnel: w424 -> [_ w437]
              tunnel: [w431 w436] -> w423
              tunnel: w422 -> [w431 w435]
              tunnel: w420 -> [_ w433]
              frame False {
              }
              frame True {
                n180 = case shown="\"NEGATIVE\", Default" "HOME LIMIT" {
                  tunnel: w437 -> [w440 w455]
                  tunnel: w435 -> [w442 w456]
                  tunnel: [w441 w457] -> w436
                  tunnel: w433 -> [w439 w454]
                  tunnel: TRUE -> [w438 w453]
                  frame "NEGATIVE", Default {
                    n181 = case shown="False" w438 {
                      tunnel: w442 -> [w446 w452]
                      tunnel: [w445 w451] -> w441
                      tunnel: w440 -> [w447 w450]
                      tunnel: w439 -> [w444 w448]
                      frame False {
                        n182 = call "FNL.vi"("System no."=w447, "Affected axes"=w444, "All axes?"=FALSE, "error in"=w446) -> ("error out"=w445:errorcluster)  [unwired: 1 in, 14 out]
                      }
                      frame True {
                        n183 = call "MNL.vi"("System no."=w450, "Affected axes"=w448, "All axes?"=FALSE, "error in"=w452) -> ("error out"=w451:errorcluster)  [unwired: 1 in, 14 out]
                      }
                    }
                  }
                  frame "POSITIVE" {
                    n184 = case shown="False" w453 {
                      tunnel: [w461 w467] -> w457
                      tunnel: w456 -> [w462 w466]
                      tunnel: w455 -> [w459 w464]
                      tunnel: w454 -> [w460 w463]
                      frame False {
                        n185 = call "FPL.vi"("System no."=w459, "Affected axes"=w460, "All axes?"=FALSE, "error in"=w462) -> ("error out"=w461:errorcluster)  [unwired: 1 in, 14 out]
                      }
                      frame True {
                        n186 = call "MPL.vi"("System no."=w464, "Affected axes"=w463, "All axes?"=FALSE, "error in"=w466) -> ("error out"=w467:errorcluster)  [unwired: 1 in, 14 out]
                      }
                    }
                  }
                }
              }
            }
            n187 = local write "PROCESS"(w418) -> ()
          }
          frame #1 {
            n188 = local write "HOME"(FALSE ("HOME")) -> ()
          }
        }
      }
      frame "HOMED ?" {
        n189 = local read "READY AXES"() -> (w483:string[])
        n190 = call "FRF?.vi"("System no."=w484, "Axes to query"=w483, "error in"=w482) -> ("Referenced?"=w476:bool[], "error out"=w481:errorcluster)  [unwired: 2 in, 13 out]
        n191 = Index Array(array=w476, index #1=0 ("index"), index #2=1 ("index"), index #3=2 ("index"), index #4=3 ("index")) -> (element #1=w474:bool, element #2=w473:bool, element #3=w472:bool, element #4=w471:bool)
        n192 = Bundle("Boolean"=w474, "Boolean"=w473, "Boolean"=w472, "Boolean"=w471) -> (→"HOMED":T16)  [unwired: 1 in]
        n193 = Compound Arithmetic op=AND(w474, w472, w473, w471) -> (w470:bool)
        "HOMED" <- w470
        n194 = shared-variable "My Computer\\PI APERTURES.lvlib\\AGGREGATE HOMED ?"(w470) -> ()  [unwired: 1 in, 1 out]
      }
      frame "WAIT FOR READY" {
        n195 = case shown="True" FALSE {
          tunnel: w489 -> [w490 w495]
          tunnel: [w490 w494] -> w488
          tunnel: w487 -> [_ w493]
          frame False {
          }
          frame True {
            n196 = local read "READY AXES"() -> (w492:string[])
            n197 = call "General wait for movement to stop.vi"("System no."=w493, "Axes to wait for"=w492, "error in"=w495, "Polling cycle \ntime, ms"=u32 500 ("Polling cycle time, ms")) -> ("error out"=w494:errorcluster)  [unwired: 14 in, 1 out]
          }
        }
        n198 = local write "PROCESS"("WAIT FOR READY" ("PROCESS")) -> ()
      }
      frame "READ RON?" {
        n199 = local read "READY AXES"() -> (w507:string[])
        n200 = call "RON?.vi"("System no."=w509, "Axes to query"=w507, "error in"=w508) -> ("Reference on?"=w505:bool[], "error out"=w506:errorcluster)  [unwired: 2 in, 13 out]
        n201 = Index Array(array=w505, index #1=0 ("index"), index #2=1 ("index"), index #3=2 ("index"), index #4=3 ("index")) -> (element #1=w500:bool, element #2=w499:bool, element #3=w498:bool, element #4=w497:bool)
        n202 = Bundle("Boolean"=w500, "Boolean"=w499, "Boolean"=w498, "Boolean"=w497) -> (→"REFER?":T16)  [unwired: 1 in]
      }
      frame "READ MIN POSITION: LIMIT OR SOFT" {
        w526 = 0.1 ("Increment")
        w527 = T17 {"Minimum"=0.0, "Maximum"=0.0, "Increment"=0.0} ("Data Entry Limits")
        w530 = TRUE ("All axes?")
        n203 = local read "READY AXES"() -> (w532:string[])
        n204 = call "TMN?.vi"("System no."=w533, "Axes to query"=w532, "All axes?"=w530, "error in"=w535) -> ("Minimum travel limit"=w534:dbl[], "error out"=w531:errorcluster)  [unwired: 1 in, 13 out]
        n205 = Index Array(array=w534) -> (element #1=w515:dbl, element #2=w514:dbl, element #3=w513:dbl, element #4=w512:dbl)  [unwired: 4 in]
        n206 = local read "STAGE MIN CLUSTER"() -> (w516:T11)
        n207 = Bundle By Name(cluster=w516, "Xo MAX"=w515, "Xm MAX"=w514, "Yo MAX"=w513, "Ym MAX"=w512) -> (w511:T11)
        "STAGE MIN CLUSTER" <- w511
        n208 = local read "STAGE MAX CLUSTER"() -> (w521:T12)
        n209 = call "TMX?.vi"("System no."=w533, "Axes to query"=w532, "All axes?"=w530, "error in"=w531) -> ("Maximum travel limit"=w528:dbl[], "error out"=w529:errorcluster)  [unwired: 1 in, 13 out]
        n210 = Index Array(array=w528) -> (element #1=w520:dbl, element #2=w519:dbl, element #3=w518:dbl, element #4=w517:dbl)  [unwired: 4 in]
        n211 = Bundle By Name(cluster=w521, "Xo MAX"=w520, "Xm MAX"=w519, "Yo MAX"=w518, "Ym MAX"=w517) -> (w510:T12)
        "STAGE MAX CLUSTER" <- w510
        n212 = shared-variable "My Computer\\PI APERTURES.lvlib\\STAGE MINIMUMS"(w511) -> ()  [unwired: 1 in, 1 out]
        n213 = Bundle(cluster=w527, "Minimum"=w515, "Maximum"=w520, "Increment"=w526) -> (w525:T17)
        n214 = Bundle(cluster=w527, "Minimum"=w513, "Maximum"=w518, "Increment"=w526) -> (w524:T17)
        n215 = Bundle(cluster=w527, "Minimum"=w514, "Maximum"=w519, "Increment"=w526) -> (w523:T17)
        n216 = Bundle(cluster=w527, "Minimum"=w512, "Maximum"=w517, "Increment"=w526) -> (w522:T17)
        n217 = property on="Xo" class="DigNum (strict)"("Data Range"=w525) -> ()  [unwired: 2 in, 2 out]
        n218 = property on="Yo" class="DigNum (strict)"("Data Range"=w524) -> ()  [unwired: 2 in, 2 out]
        n219 = property on="Xm" class="DigNum (strict)"("Data Range"=w523) -> ()  [unwired: 2 in, 2 out]
        n220 = property on="Ym" class="DigNum (strict)"("Data Range"=w522) -> ()  [unwired: 2 in, 2 out]
        n221 = shared-variable "My Computer\\PI APERTURES.lvlib\\STAGE MAXIMUMS"(w510) -> ()  [unwired: 1 in, 1 out]
      }
      frame "READ STAGE LIMIT SWITCHES " {
        n222 = local read "READY AXES"() -> (w546:string[])
        n223 = call "LIM?.vi"("System no."=w549, "Axes to query"=w546, "error in"=w548) -> ("Axis with limit switch?"=w537:bool[], "error out"=w547:errorcluster)  [unwired: 2 in, 13 out]
        n224 = Index Array(array=w537, index #1=0 ("index"), index #2=1 ("index"), index #3=2 ("index"), index #4=3 ("index")) -> (element #1=w541:bool, element #2=w540:bool, element #3=w539:bool, element #4=w538:bool)
        n225 = Bundle("Boolean"=w541, "Boolean"=w540, "Boolean"=w539, "Boolean"=w538) -> (→"LIMITS ?":T16)  [unwired: 1 in]
      }
      frame "GOTO POSITION" {
        n226 = local read "SET APERTURE"() -> (w555:cluster{"Xm":dbl, "Ym":dbl})
        n227 = local read "SET POSITION"() -> (w556:T1)
        n228 = flat-sequence {
          tunnel: w561 -> [w567]
          tunnel: w559 -> [w565]
          tunnel: [w566] -> w557
          tunnel: w550 -> [w562]
          tunnel: [w570] -> w560
          tunnel: w557 -> [w570]
          frame #0 {
            n229 = local read "READY AXES"() -> (w564:string[])
            n230 = call "MOV.vi"("System no."=w565, "Axes to move"=w564, "Position values"=w562, "No.of digits"=i16 4, "error in"=w567) -> ("error out"=w566:errorcluster)  [unwired: 14 in]
          }
          frame #1 {
            n231 = local write "OUT (+)"(FALSE ("OUT (+)")) -> ()
            n232 = local write "IN (-)"(FALSE ("IN (-)")) -> ()
          }
        }
        n233 = Unbundle(w556) -> ("Xo"=w554:dbl, "Yo"=w553:dbl)
        n234 = Unbundle(w555) -> ("Xm"=w552:dbl, "Ym"=w551:dbl)
        n235 = Build Array(w554, w552, w553, w551) -> (w550:dbl[])
        n236 = local write "PROCESS"("GOTO POINT" ("PROCESS")) -> ()
      }
      frame "SET POSITION" {
        n237 = local read "STAGE MAX CLUSTER"() -> (w578:T12)
        n238 = local read "STAGE MIN CLUSTER"() -> (w579:T11)
        n239 = local read "HOME LIMIT"() -> (w580:enum16{"NEGATIVE", "POSITIVE"})
        n240 = local read "HOME AXES"() -> (w581:enum16{"1 & 2", "3 & 4"})
        n241 = case shown="\"1 & 2\", Default" w581 {
          tunnel: w580 -> [w589 w596]
          tunnel: w579 -> [w588 w601]
          tunnel: w578 -> [w587 w600]
          tunnel: [w586 w599] -> w575
          tunnel: [w585 w598] -> w574
          tunnel: [string[] ["1", "2"] string[] ["3", "4"]] -> w571
          frame "1 & 2", Default {
            n242 = case shown="\"POSITIVE\"" w589 {
              tunnel: w588 -> [w592 _]
              tunnel: w587 -> [_ w595]
              tunnel: [w591 w594] -> w586
              tunnel: [w590 w593] -> w585
              frame "NEGATIVE", Default {
                n243 = Unbundle By Name(w592) -> ("Xo MAX"=w591:dbl, "Xm MAX"=w590:dbl)
              }
              frame "POSITIVE" {
                n244 = Unbundle By Name(w595) -> ("Xo MAX"=w594:dbl, "Xm MAX"=w593:dbl)
              }
            }
          }
          frame "3 & 4" {
            n245 = case shown="\"POSITIVE\"" w596 {
              tunnel: w601 -> [w604 _]
              tunnel: w600 -> [_ w607]
              tunnel: [w603 w606] -> w599
              tunnel: [w602 w605] -> w598
              frame "NEGATIVE", Default {
                n246 = Unbundle By Name(w604) -> ("Yo MAX"=w603:dbl, "Ym MAX"=w602:dbl)
              }
              frame "POSITIVE" {
                n247 = Unbundle By Name(w607) -> ("Yo MAX"=w606:dbl, "Ym MAX"=w605:dbl)
              }
            }
          }
        }
        n248 = Build Array(w575, w574) -> (w573:dbl[])
        n249 = local write "PROCESS"("SET POINT VALUES" ("PROCESS")) -> ()
        n250 = call "POS.vi"("System no."=w583, "Axes to set"=w571, "Position values"=w573, "No.of digits"=i16 4, "error in"=w582) -> ("error out"=w577:errorcluster)  [unwired: 14 out]
      }
      frame "READ POSITION" {
        n251 = local read "HOMED"() -> (w610:bool)
        n252 = case shown="True" w610 {
          tunnel: w613 -> [_ w633]
          tunnel: w612 -> [w615 w632]
          tunnel: [w615 w631] -> w611
          tunnel: [w614 w617] -> w609
          tunnel: [w614 w617] -> w608
          frame False {
            w614 = FALSE
          }
          frame True {
            w617 = TRUE
            n253 = local read "READY AXES"() -> (w625:string[])
            n254 = First Call?() -> (First Call?: T/F=w616:bool)
            n255 = call "POS?.vi"("System no."=w633, "Axes to query"=w625, "error in"=w632) -> ("Position"=w630:dbl[], "error out"=w631:errorcluster)  [unwired: 2 in, 13 out]
            n256 = case shown="True" w616 {
              frame False {
              }
              frame True {
                n257 = local read "APERTURE POSITION"() -> (w635:cluster{"Xm":dbl, "Ym":dbl})
                n258 = local read "OBJECT POSITION"() -> (w634:T1)
                n259 = local write "SET POSITION"(w634) -> ()
                n260 = local write "SET APERTURE"(w635) -> ()
              }
            }
            n261 = Index Array(array=w630, index #1=0 ("index"), index #2=1 ("index"), index #3=2 ("index"), index #4=3 ("index")) -> (element #1=w623:dbl, element #2=w619:dbl, element #3=w622:dbl, element #4=w618:dbl)
            n262 = local read "OBJECT POSITION"() -> (w621:T1)
            n263 = Bundle(cluster=w621, "Xo"=w623, "Yo"=w622) -> (→"OBJECT POSITION":T1)
            n264 = Bundle(cluster=w621, "Xo"=w619, "Yo"=w618) -> (→"APERTURE POSITION":T1)
          }
        }
        n265 = property on="APERTURE POSITION" class="Clust (strict)"("Visible"=w608) -> ()  [unwired: 2 in, 2 out]
        n266 = property on="OBJECT POSITION" class="Clust (strict)"("Visible"=w609) -> ()  [unwired: 2 in, 2 out]
      }
      frame "READ SERVO SETTINGS" {
        # "read default values"
        n267 = Build Array(10 ("element"), 1 ("element"), 2 ("element"), 3 ("element")) -> (w656:i32[])
        n268 = call "SPA?.vi"("System no."=w643, "Parameter no."=w656, "error in"=w642) -> ("Parameter value"=w652:dbl[], "error out"=w655:errorcluster)  [unwired: 4 in, 11 out]
        n269 = call "VEL?.vi"("System no."=w643, "error in"=w655) -> ("Velocity"=w654:dbl[], "error out"=w641:errorcluster)  [unwired: 3 in, 13 out]
        n270 = Index Array(array=w652, index=1) -> (element=w638:dbl)
        n271 = Index Array(array=w652, index=2) -> (element=w637:dbl)
        n272 = Index Array(array=w652, index=3) -> (element=w636:dbl)
        n273 = Index Array(array=w654, index=0) -> (element=w653:dbl)
        n274 = local write "VELOCITY"(w653) -> ()
        n275 = local read "SERVO PID"() -> (w639:cluster{"P":dbl, "I":dbl, "D":dbl})
        n276 = Bundle By Name(cluster=w639, "P"=w638, "I"=w637, "D"=w636) -> (w640:cluster{"P":dbl, "I":dbl, "D":dbl})
        n277 = local write "SERVO PID"(w640) -> ()
      }
      frame "SET SERVO PID" {
        n278 = local read "SERVO PID"() -> (w660:cluster{"P":dbl, "I":dbl, "D":dbl})
        n279 = Unbundle By Name(w660) -> ("P"=w659:dbl, "I"=w658:dbl, "D"=w657:dbl)
        n280 = Build Array(w659, w658, w657) -> (w669:dbl[])
        n281 = Build Array(1 ("element"), 2 ("element"), 3 ("element")) -> (w668:i32[])
        n282 = call "SPA.vi"("System no."=w662, "Axis to set"=string[] ["1", "2", "3"], "Parameter value"=w669, "error in"=w664, "Parameter number"=w668) -> ("error out"=w663:errorcluster)  [unwired: 5 in, 9 out]
      }
      frame "SET SERVO MOTORS ON" {
        n283 = local read "READY AXES"() -> (w670:string[])
        n284 = call "SVO.vi"("System no."=w672, "Axes to command"=w670, "Servo mode"=bool[] [TRUE, TRUE, TRUE, TRUE], "error in"=w673) -> ("error out"=w671:errorcluster)  [unwired: 1 in, 14 out]
      }
      frame "SET VELOCITIES" {
        n285 = local read "READY AXES"() -> (w675:string[])
        n286 = local read "VELOCITY"() -> (w679:dbl)
        n287 = Build Array(w679) -> (w680:dbl[])
        n288 = call "VEL.vi"("System no."=w678, "Axes to set"=w675, "Velocity values"=w680, "error in"=w676) -> ("error out"=w677:errorcluster)  [unwired: 2 in, 13 out]
      }
      frame "CLR ERRORS" {
        n289 = Unbundle By Name(w685) -> ("code"=w689:i32)
        n290 = local read "READY AXES"() -> (w682:string[])
        n291 = Equal?(x=5 ("y"), y=w689) -> (x = y?=w688:bool)
        n292 = Equal?(x=w689, y=-1024) -> (x = y?=w686:bool)
        n293 = Or(x=w688, y=w686) -> (x .or. y?=w687:bool)
        n294 = case shown="True" w687 {
          tunnel: [errorcluster {"status"=FALSE, "code"=0, "source"=""} ("error out") w696] -> w684
          tunnel: w683 -> [_ w695]
          tunnel: w682 -> [_ w694]
          frame False {
          }
          frame True {
            n295 = call "CLR.vi"("System no."=w695, "CLR axes"=w694, "All axes?"=FALSE) -> ("error out"=w697:errorcluster)  [unwired: 2 in, 14 out]
            n296 = call "ERR?.vi"("System no."=w695, "error in"=w697) -> ("error out"=w696:errorcluster)  [unwired: 17 out]
          }
        }
        n297 = local write "PROCESS"("CLEARING ERRORS !" ("PROCESS")) -> ()
      }
    }
    n298 = case shown="Error" w304 {
      selector: w304 -> [w310 w319]
      tunnel: w303 -> [w311 w321]
      tunnel: [w311 w320] -> w302
      tunnel: [w310 w318] -> w301
      frame No Error {
      }
      frame Error {
        n299 = flat-sequence {
          tunnel: w319 -> [w327]
          tunnel: w321 -> [w328]
          tunnel: [w328] -> w314
          tunnel: [w327] -> w313
          tunnel: [w323] -> w312
          tunnel: [w334] -> w317
          tunnel: [w333] -> w316
          tunnel: [w332] -> w315
          tunnel: w314 -> [w334]
          tunnel: w313 -> [w333]
          tunnel: w312 -> [w329]
          tunnel: [w338] -> w320
          tunnel: [w336] -> w318
          tunnel: w317 -> [w339]
          tunnel: w316 -> [w337]
          tunnel: w315 -> [w335]
          frame #0 {
            n300 = Unbundle(w327) -> ("code"=w326:i32)  [unwired: 2 out]
            n301 = Number To Decimal String(number=w326) -> (decimal integer string=w324:string)  [unwired: 1 in]
            n302 = Concatenate Strings("Clear Error  " ("message"), w324, "?" ("string")) -> (w323:string)
          }
          frame #1 {
            n303 = Two Button Dialog(message=w329, 1:"No" ("F button name (\"Cancel\")"), 2:"Yes" ("T button name (\"OK\")")) -> (T button?=w332:bool)
          }
          frame #2 {
            n304 = case shown="False" w335 {
              selector: w335 -> [w341 _]
              tunnel: w339 -> [w343 w348]
              tunnel: [w343 w347] -> w338
              tunnel: w337 -> [w342 w345]
              tunnel: [w342 w344] -> w336
              frame False {
                n305 = Not(x=w341) -> (.not. x?=w340:bool)
                n306 = Stop(stop? (T)=w340) -> ()
              }
              frame True {
                n307 = Enqueue Element(queue=w348, element=APERTURE_EVENTS."CLR ERRORS", error in (no error)=w345) -> (queue out=w347:refnum<queue>, error out=w344:errorcluster)  [unwired: 1 in, 1 out]
              }
            }
          }
        }
      }
    }
    n308 = local write "error out"(w304) -> ()
    n309 = local read "stop"() -> (w307:bool)
  }
  n310 = call "ERR?.vi"("System no."=w5, "error in"=w8) -> ("error out"=w17:errorcluster)  [unwired: 17 out]
  n311 = call "GCSTranslateError.vi"("error in"=w17) -> ("error out"=w16:errorcluster)  [unwired: 18 out]
  n312 = call "Close connection if open.vi"("System no."=w5, "error in"=w16) -> ("error out"=→"error out":errorcluster)  [unwired: 1 in, 16 out]
